vi "2.vi"() -> ()   [LabVIEW 2017]
panel:
  in  "停止":bool
  in  "旋钮":dbl(knob) scale=0.2..1.0
  out "布尔 5":bool
  out "布尔 4":bool
  out "布尔 3":bool
  out "布尔 2":bool
  out "布尔":bool
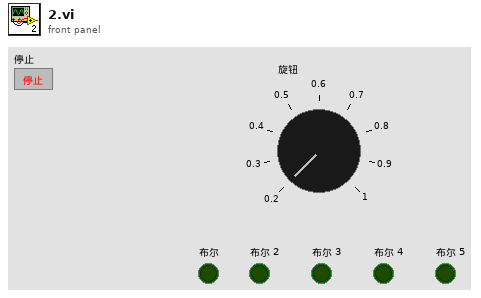
[diagram p1: front panel]
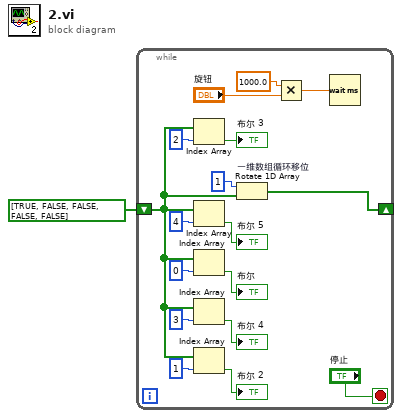
[diagram p0: block diagram]
diagram:
  n1 = while {
    shift-right: [w17] -> _
    shift-left: bool[] [TRUE, FALSE, FALSE, FALSE, FALSE] -> [w14]
    stop <- "停止" stop-if-true
    n2 = Index Array(array=w14, index=2 ("索引")) -> (element=→"布尔 3":bool)
    n3 = Index Array(array=w14, index=4 ("索引")) -> (element=→"布尔 5":bool)
    n4 = Index Array(array=w14, index=0 ("索引")) -> (element=→"布尔":bool)
    n5 = Index Array(array=w14, index=3 ("索引")) -> (element=→"布尔 4":bool)
    n6 = Index Array(array=w14, index=1 ("索引")) -> (element=→"布尔 2":bool)
    n7 = Rotate 1D Array "一维数组循环移位"(1:w14, 2:1 ("n")) -> (0:w17:bool[])
    n8 = Multiply(x=1000.0, y="旋钮") -> (x*y=w2:dbl)
    n9 = Wait (ms)(milliseconds to wait=w2) -> ()  [unwired: 1 out]
  }
